vi "InitRobot.vi"(7 "Camera Name":refnum<k21>="cam0" caption="IMAQdx Session", 8 "VISA resource name":refnum<visa-resource-name>, 9 "input cluster":T1={"New Image"=refnum, "Session Out"="", "LIDAR VISA Name"="", "Phidget Device Out"=0, "Lidar Data"=[], "polar attributes"={"maximum"=0.0, "minimum"=0.0, "clip to min"=FALSE, "log?(F)"=FALSE, "grid color"=6710886, "plot color"=65280, "fmt and prec"={"format"=enum."Decimal", "precision"=0}, "visible section"=8}, "Debug Message"="", "Servo Angles"={"Angle X"=0.0, "Angle Y"=0.0}, "ColorPlane"=refnum, "Threshold"=refnum, "PartFilt"=refnum, "Processed Image"=refnum, "Magnitude"=[], "Direction"=[]} {"polar attributes"."minimum" format="%0.2f"; "polar attributes"."maximum" format="%0.2f"}) -> (3 "input cluster 2":T1={"New Image"=refnum, "Session Out"="", "LIDAR VISA Name"="", "Phidget Device Out"=0, "Lidar Data"=[], "polar attributes"={"maximum"=0.0, "minimum"=0.0, "clip to min"=FALSE, "log?(F)"=FALSE, "grid color"=6710886, "plot color"=65280, "fmt and prec"={"format"=enum."Decimal", "precision"=0}, "visible section"=8}, "Debug Message"="", "Servo Angles"={"Angle X"=0.0, "Angle Y"=0.0}, "ColorPlane"=refnum, "Threshold"=refnum, "PartFilt"=refnum, "Processed Image"=refnum, "Magnitude"=[], "Direction"=[]} {"polar attributes"."minimum" format="%0.2f"; "polar attributes"."maximum" format="%0.2f"}, 5 "error out":errorcluster)   [LabVIEW 2014]
uses:
  controls/Data.ctl
  <vilib>/vision/Image Controls.llb/IMAQ Image.ctl
  <vilib>/userdefined/High Color/IMAQdx.ctl
  Program Files (x86)/National Instruments/LabVIEW 2014/instr.lib/Hokuyo URG Series/Public/Initialize-Standard.vi
  <vilib>/vision/driver/NI_Vision_Acquisition_Software.lvlib
  Program Files (x86)/National Instruments/LabVIEW 2014/instr.lib/Hokuyo URG Series/Hokuyo URG Series.lvlib
panel:
  out "VISA resource name out":refnum<visa-resource-name>
  out "Device Out":i32
  # "LIDAR I/O"
  # "Camera I/O"
  # "Phidget I/O"
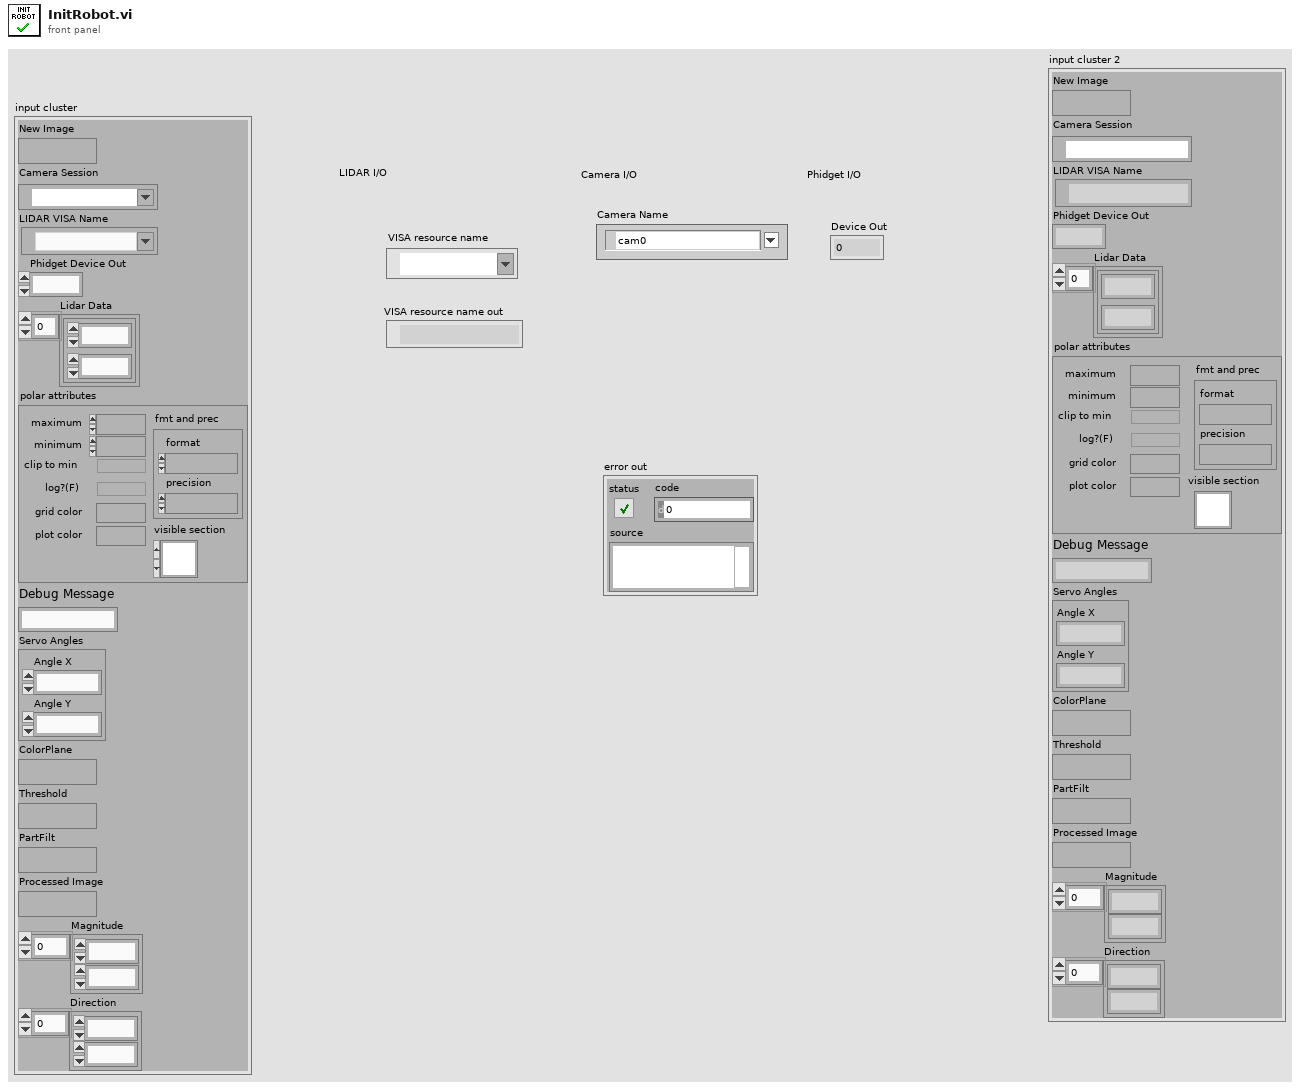
[diagram p1: front panel]
types:
  T1 = typedef "Data.ctl" = cluster{"New Image":T2, "Session Out":T3, "LIDAR VISA Name":refnum<visa-resource-name>, "Phidget Device Out":i32, "Lidar Data":cluster{dbl, dbl}[], "polar attributes":cluster{"maximum":dbl, "minimum":dbl, "clip to min":bool, "log?(F)":bool, "grid color":u32, "plot color":u32, "fmt and prec":cluster{"format":enum8{"Decimal", "Scientific", "Engineering", "Binary", "Octal", "Hex"}, "precision":u8}, "visible section":u16}, "Debug Message":string, "Servo Angles":cluster{"Angle X":dbl, "Angle Y":dbl}, "ColorPlane":T2, "Threshold":T2, "PartFilt":T2, "Processed Image":T2, "Magnitude":dbl[], "Direction":dbl[]}
  T2 = typedef "IMAQ Image.ctl" = refnum<image>
  T3 = typedef "IMAQdx.ctl" = refnum<k21>
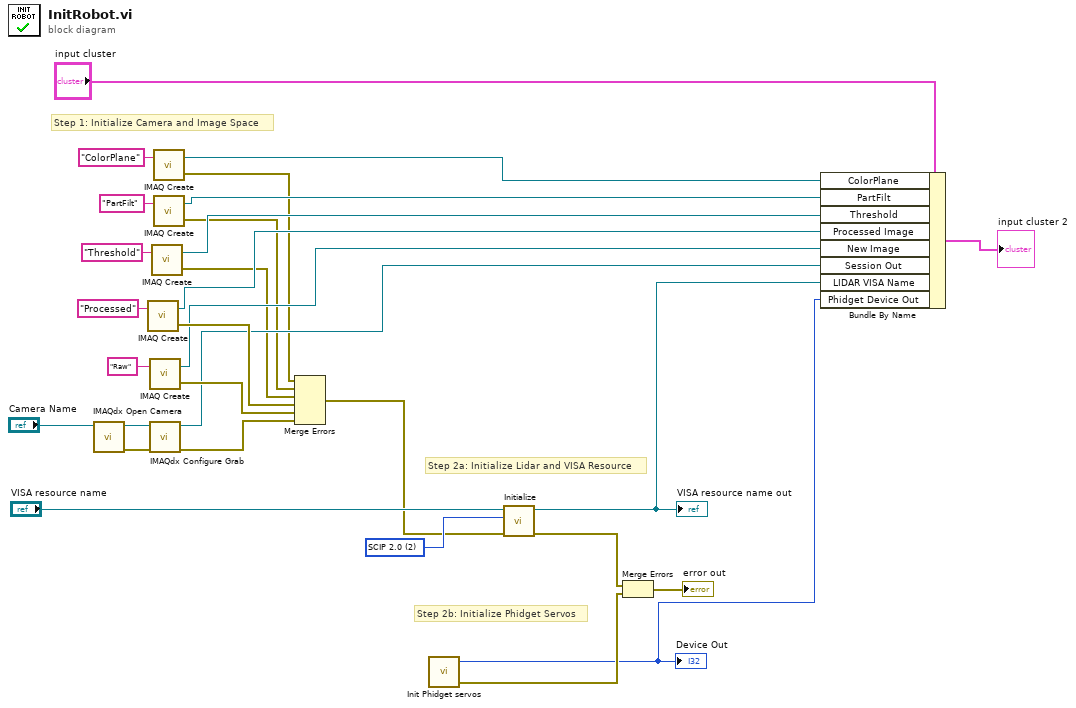
[diagram p0: block diagram]
diagram:
  w23 = u32 2 items=["Convert to Latest", "SCIP 1.1", "SCIP 2.0"] ("Protocol")
  # "Step 2b: Initialize Phidget Servos"
  # "Step 2a: Initialize Lidar and VISA Resource"
  # "Step 1: Initialize Camera and Image Space"
  n1 = call <vilib>:"IMAQdx Open Camera.vi"("Session In"="Camera Name") -> ("error out"=w27:errorcluster, "Session Out"=w28:T3)  [unwired: 2 in, 7 out]
  n2 = call "IMAQ Create"("Image Name"="Processed") -> ("New Image"=w10:T2, "error out"=w17:errorcluster)  [unwired: 3 in, 1 out]
  n3 = call "IMAQ Create"("Image Name"="Raw") -> ("New Image"=w9:T2, "error out"=w26:errorcluster)  [unwired: 3 in, 1 out]
  n4 = call <vilib>:"IMAQdx Configure Grab.vi"("error in"=w27, "Session In"=w28) -> ("error out"=w25:errorcluster, "Session Out"=w8:T3)  [unwired: 8 out]
  n5 = call "IMAQ Create"("Image Name"="Threshold") -> ("New Image"=w11:T2, "error out"=w4:errorcluster)  [unwired: 3 in, 1 out]
  n6 = call "IMAQ Create"("Image Name"="ColorPlane") -> ("New Image"=w1:T2, "error out"=w2:errorcluster)  [unwired: 3 in, 1 out]
  n7 = call "IMAQ Create"("Image Name"="PartFilt") -> ("New Image"=w12:T2, "error out"=w5:errorcluster)  [unwired: 3 in, 1 out]
  n8 = Merge Errors(w2, w5, w4, w17, w26, w25) -> (w22:errorcluster)
  n9 = call "Init Phidget servos.vi"() -> ("Device Out"=w6:i32, "error out"=w20:errorcluster)  [unwired: 1 in, 1 out]
  "Device Out" <- w6
  n10 = call-poly "Initialize.vi"("error in (no error)"=w22, "Protocol (2: SCIP 2.0)"=w23, "VISA resource name"="VISA resource name") -> ("error out"=w21:errorcluster, "VISA resource name out"=w7:refnum<visa-resource-name>)  [unwired: 7 in]
  "VISA resource name out" <- w7
  n11 = Merge Errors(w21, w20) -> (→"error out":errorcluster)
  n12 = Bundle By Name(cluster="input cluster", "ColorPlane"=w1, "PartFilt"=w12, "Threshold"=w11, "Processed Image"=w10, "New Image"=w9, "Session Out"=w8, "LIDAR VISA Name"=w7, "Phidget Device Out"=w6) -> (→"input cluster 2":T1)
